vi "WaveformGraph.vi"() -> ()   [LabVIEW 2018]
panel:
  out "Array":dbl[](array[numeric])
  out "Waveform Graph":dbl[](graph)
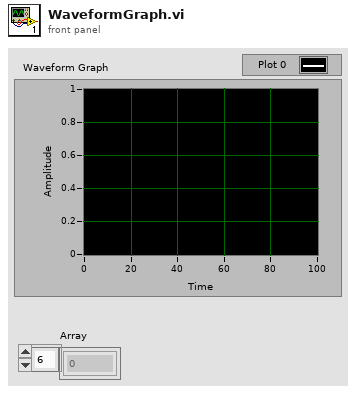
[diagram p1: front panel]
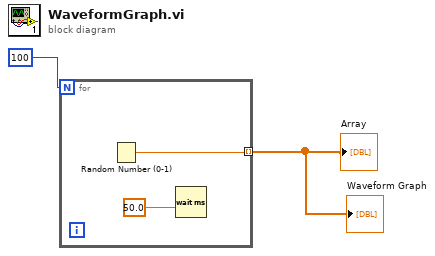
[diagram p0: block diagram]
diagram:
  n1 = for {
    N: 100 -> [_]
    tunnel: [w4] -> w1 mode=indexing
    n2 = Random Number (0-1)() -> (number: 0 to 1=w4:dbl)
    n3 = Wait (ms)(milliseconds to wait=50.0) -> ()  [unwired: 1 out]
  }
  "Waveform Graph" <- w1
  "Array" <- w1
